vi "Scale Data.vi"(10 "Raw Graph Data":T3, 11 "Channel Settings":T1[](array[typedef])) -> (2 "Scaled Graph Data":T3)   [LabVIEW 2021, in "Acquisition.lvlib"]
doc: "Use the Calibration Information from 'Channel Settings' to scale the 'Raw Graph Data' and return it in 'Scaled Graph Data'."
uses:
  Acquisition.lvlib
  controls/Acquired Data.ctl
  Channel Settings.ctl
  IO Device.ctl
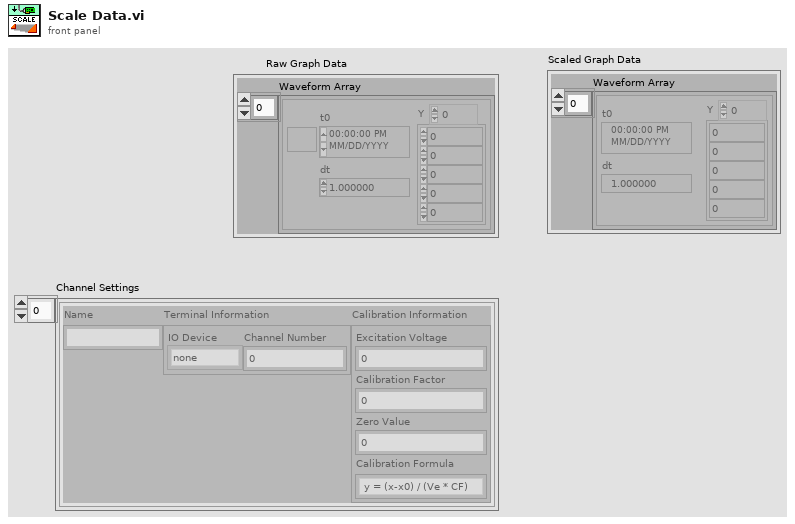
[diagram p1: front panel]
types:
  T1 = typedef "Acquisition.lvlib/Channel Settings.ctl" = cluster{"Name":string, "Terminal Information":cluster{"IO Device":T2, "Channel Number":i32}, "Calibration Information":cluster{"Excitation Voltage":dbl, "Calibration Factor":dbl, "Zero Value":dbl, "Calibration Formula":string}}
  T2 = typedef "Acquisition.lvlib/IO Device.ctl" = enum16{"none", "9219", "9401"}
  T3 = typedef "Acquired Data.ctl" = cluster{"Waveform Array":waveform(dbl)[]}
  T4 = cluster{"Excitation Voltage":dbl, "Calibration Factor":dbl, "Zero Value":dbl, "Calibration Formula":string}
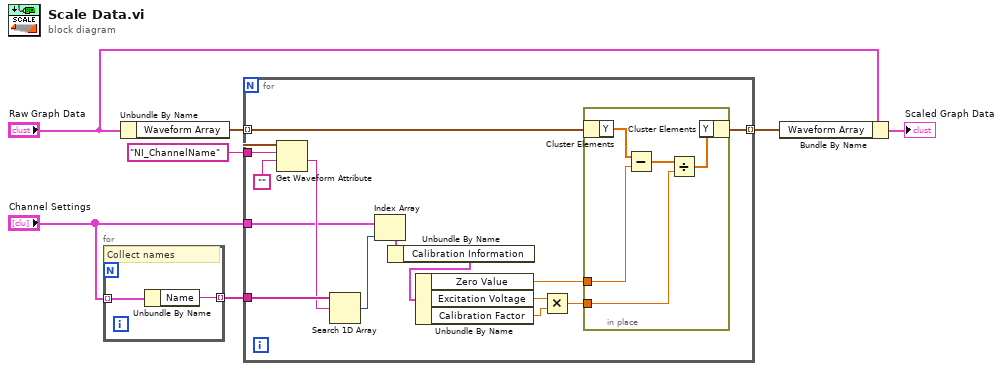
[diagram p0: block diagram]
diagram:
  n1 = for {
    tunnel: "Channel Settings" -> [w9] mode=indexing
    tunnel: [w8] -> w2 mode=indexing
    # "Collect names"
    n2 = Unbundle By Name(w9) -> ("Name"=w8:string)
  }
  n3 = Unbundle By Name("Raw Graph Data") -> ("Waveform Array"=w7:waveform(dbl)[])
  n4 = for {
    tunnel: w7 -> [w23] mode=indexing
    tunnel: "NI_ChannelName" ("name") -> [w22]
    tunnel: [w21] -> w3 mode=indexing
    tunnel: w2 -> [w19]
    tunnel: "Channel Settings" -> [w17]
    n5 = Get Waveform Attribute(5:"", 6:w22, 7:w23) -> (1:w18:string)  [unwired: 1 in, 3 out]
    n6 = Search 1D Array(1D array=w19, element=w18) -> (index of element=w16:i32)  [unwired: 1 in]
    n7 = Index Array(array=w17, index=w16) -> (element=w15:T1)
    n8 = Unbundle By Name(w15) -> ("Calibration Information"=w14:T4)
    n9 = Unbundle By Name(w14) -> ("Zero Value"=w10:dbl, "Excitation Voltage"=w13:dbl, "Calibration Factor"=w12:dbl)
    n10 = Multiply(x=w13, y=w12) -> (x*y=w11:dbl)
    n11 = in-place {
      in-place-border: w11 -> [w25]
      in-place-border: w10 -> [w27]
      n12 = in-place-cluster #1(w23) -> ("Y"=w28:dbl[])
      n13 = Subtract(x=w28, y=w27) -> (x-y=w26:dbl[])
      n14 = Divide(x=w26, y=w25) -> (x/y=w24:dbl[])
      n15 = in-place-cluster #1("Y"=w24) -> (w21:waveform(dbl))
    }
  }
  n16 = Bundle By Name(cluster="Raw Graph Data", "Waveform Array"=w3) -> (→"Scaled Graph Data":T3)
